vi "PDash Validate Module.vi"(8 "error in":errorcluster, 10 "Current Selection":T1, 11 "Project":refnum<class "Project.lvclass">) -> (0 "error out":errorcluster, 3 "Project Out":refnum<class "Project.lvclass">)   [LabVIEW 2020, in "Panther Dashboard.lvlib"]
doc: "Panther Dashboard DQMH UI Template"
uses:
  Panther Dashboard.lvlib
  Class/Project/Project.lvclass
  C:/GitClones/PantherDashboard/src/LabVIEW/Panther Dashboard/Class/LabVIEWItem/LabVIEWItem.lvclass
  Class/Library/Library.lvclass
  Class/VI/VI.lvclass
  Class/Library/Library.lvclass/Library.ctl
  Class/LabVIEWItem/LabVIEWItem.lvclass/LabVIEWItem.ctl
  Class/Project/Project.lvclass/Project.ctl
  Class/Library/Read Library Ref.vi
  Class/LabVIEWItem/Read Item Name.vi
  Class/Project/Read Main App Inst Ref.vi
  Class/LabVIEWItem/Read Item Path.vi
  Class/Project/Read Target Ref.vi
  Class/Project/Read Project Ref.vi
  Class/LabVIEWItem/Write Item Description.vi
  Class/Project/Write Project Ref.vi
  Class/LabVIEWItem/Write Item Name.vi
  Class/Project/Write Target Name.vi
  Class/Project/Write Target Ref.vi
  Class/Project/Write Target App Ins Ref.vi
  Class/Project/Write Main App Inst Ref.vi
  Class/LabVIEWItem/Write Item Path.vi
  Class/LabVIEWItem/Write Item Type.vi
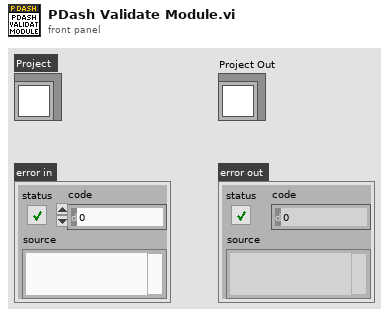
[diagram p1: front panel]
types:
  T1 = cluster{"Library":refnum<class "Library.lvclass">, "VI":refnum<class "VI.lvclass">}
  T2 = typedef "DQMH Validate Module.lvlib/Validation Result.ctl" = cluster{"Test Result":T3, "Issue Text":string, "Category Text":string, "Details Message":string, "Fixer VI":path, "Error":errorcluster, "Data for Fixer":variant, "Library":refnum<vi>, "Double Click VI":path, "Data for Double Click":variant}
  T3 = typedef "DQMH Validate Module.lvlib/Test Result.ctl" = enum16{"Pass", "Fail", "Error"}
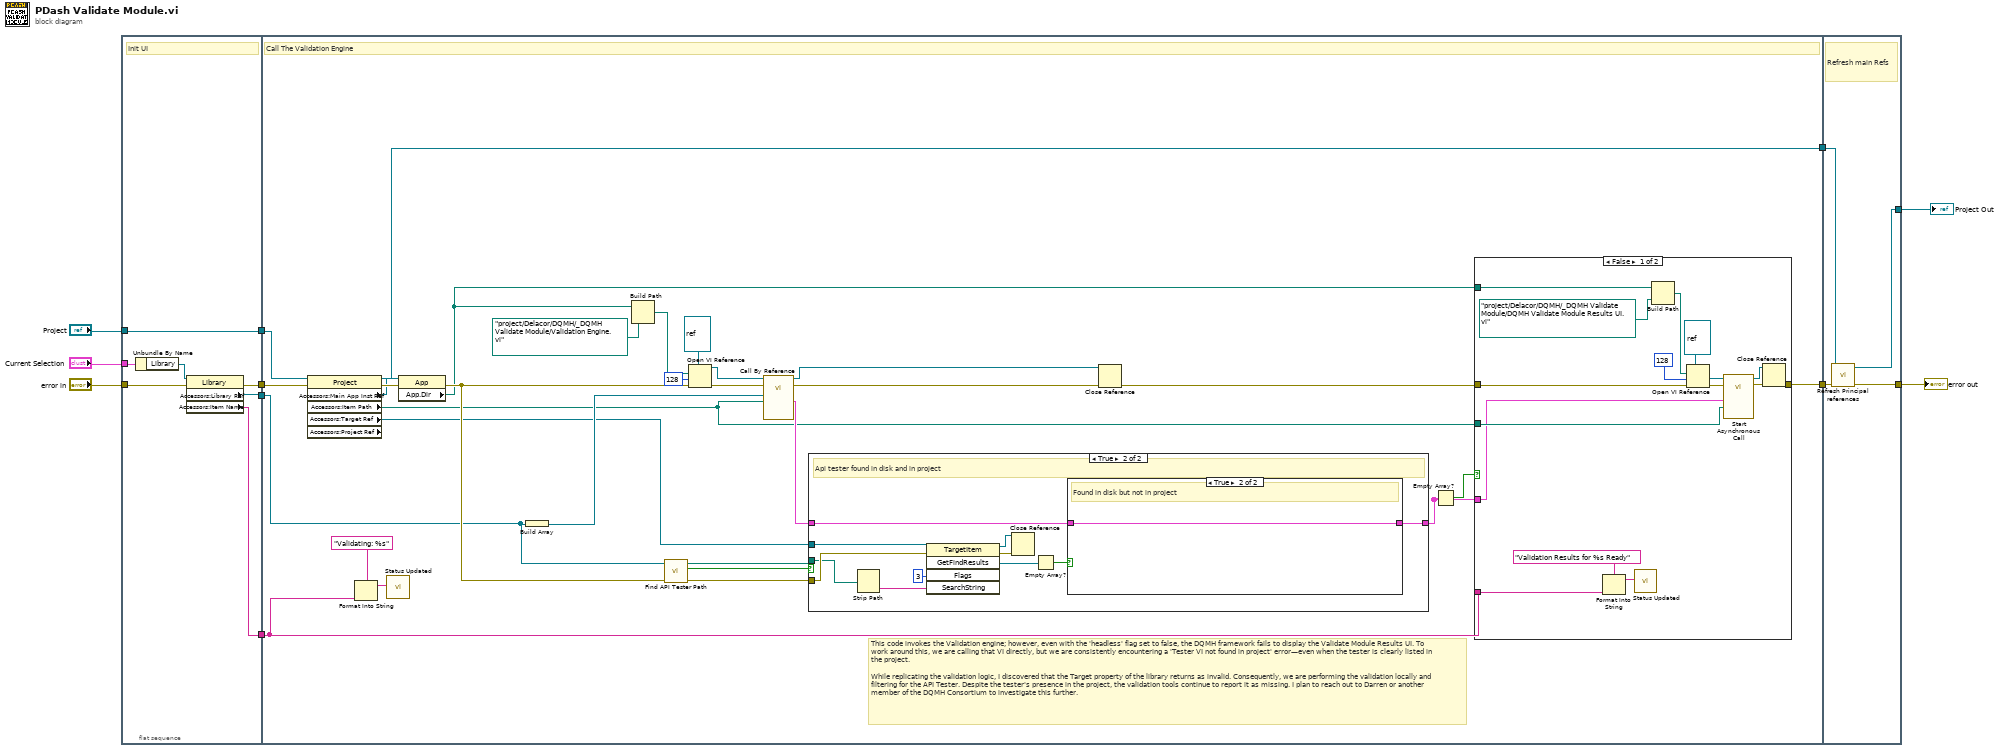
[diagram p0: block diagram]
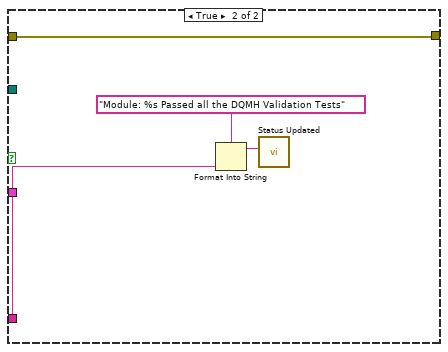
[diagram p2: hidden frame]
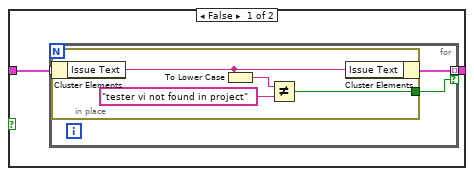
[diagram p4: hidden frame]
diagram:
  n1 = flat-sequence {
    tunnel: "Project" -> [w16]
    tunnel: [w16] -> w6
    tunnel: "error in" -> [w18]
    tunnel: [w17] -> w8
    tunnel: "Current Selection" -> [w15]
    tunnel: [w13] -> w4
    tunnel: [w12] -> w3
    tunnel: [w44] -> w11
    tunnel: w6 -> [w40]
    tunnel: w8 -> [w48]
    tunnel: w4 -> [w28]
    tunnel: w3 -> [w23]
    tunnel: [w19] -> w2
    tunnel: [w93] -> w10
    tunnel: w11 -> [w94]
    tunnel: w2 -> [w92]
    tunnel: [w91] -> w1
    frame #0 {
      # "Init UI"
      n2 = Unbundle By Name(w15) -> ("Library"=w14:refnum<class "Library.lvclass">)
      n3 = property class="Library"(reference=w14, error in=w18) -> (error out=w17:errorcluster, "Accessors:Library Ref"=w13:refnum<vi>, "Accessors:Item Name"=w12:string)  [unwired: 1 out]
    }
    frame #1 {
      # "This code invokes the Validation engine; however, even with the 'headless' flag set to false, the DQMH framework fails to display the Validate Module Results UI. To work around this, we are calling that VI directly, but we are consistently encountering a 'Tester VI not found in project' error—even when the tester is clearly listed in the project.\n\nWhile replicating the validation logic, I discovered that the Target property of the library returns as invalid. Consequently, we are performing the validation locally and filtering for the API Tester. Despite the tester's presence in the project, the validation tools continue to report it as missing. I plan to reach out to Darren or another member of the DQMH Consortium to investigate this further."
      # "Call The Validation Engine"
      n4 = property class="Project" props=["Accessors:Main App Inst Ref", "Accessors:Item Path", "Accessors:Target Ref", "Accessors:Project Ref"](reference=w40, error in=w48) -> (reference out=w19:refnum<class "Project.lvclass">, error out=w47:errorcluster, "Accessors:Main App Inst Ref"=w39:refnum<vi>, "Accessors:Item Path"=w26:path, "Accessors:Target Ref"=w20:refnum<vi>)  [unwired: 1 out]
      n5 = Format Into String(format string="Validating: %s" ("Status"), w23) -> (resulting string=w34:string)  [unwired: 2 in, 1 out]
      n6 = call "Status Updated.vi"("Status"=w34) -> ()  [unwired: 10 in, 1 out]
      n7 = property class="App"(reference=w39, error in=w47) -> (error out=w42:errorcluster, "App.Dir"=w31:path)  [unwired: 1 out]
      n8 = Build Array(w28) -> (w35:refnum<vi>[])
      n9 = Build Path(base path=w31, name or relative path=path "project/Delacor/DQMH/_DQMH Validate Module/Validation Engine.vi") -> (appended path=w38:path)
      n10 = call "Find API Tester Path.vi"("error in"=w42, "DQMH Library Ref"=w28) -> ("error out"=w41:errorcluster, "Api tester found?"=w22:bool, "API Tester Path"=w21:path)  [unwired: 7 in]
      n11 = Open VI Reference(type specifier VI Refnum (for type only)=refnum<vi> refnum, vi path=w38, options=128, error in (no error)=w42) -> (vi reference=w32:refnum<vi>, error out=w43:errorcluster)  [unwired: 2 in]
      n12 = call-by-ref "?"(reference=w32, error in=w43, "Project Path"=w26, "Libraries in"=w35) -> (reference out=w30:refnum<vi>, error out=w46:errorcluster, "Validation Results"=w27:T2[])  [unwired: 6 in, 3 out]
      n13 = case shown="True" w22 {
        tunnel: w27 -> [w69 w78]
        tunnel: [w69 w77] -> w25
        tunnel: w41 -> [_ w79]
        tunnel: w21 -> [_ w73]
        tunnel: w20 -> [_ w72]
        frame False {
          # "Api Tester Not found in project"
        }
        frame True {
          # "Api tester found in disk and in project"
          n14 = Strip Path(path=w73) -> (name=w75:string)  [unwired: 1 out]
          n15 = invoke class="TargetItem" method="GetFindResults"(reference=w72, error in=w79, "Flags"=3, "SearchString"=w75) -> (reference out=w70:refnum<vi>, error out=w80:errorcluster, "GetFindResults"=w74:refnum<vi>[])  [unwired: 1 in, 2 out]
          n16 = Close Reference(reference=w70, error in (no error)=w80) -> ()  [unwired: 1 out]
          n17 = Empty Array?(array=w74) -> (empty?=w71:bool)
          n18 = case shown="True" w71 {
            tunnel: w78 -> [w82 w90]
            tunnel: [w81 w90] -> w77
            frame False {
              n19 = for {
                tunnel: w82 -> [w85] mode=indexing
                tunnel: [w84] -> w81 mode=indexing if=w83
                n20 = in-place {
                  in-place-border: [w87] -> w83
                  n21 = in-place-cluster #1(w85) -> ("Issue Text"=w88:string)
                  n22 = To Lower Case(string=w88) -> (all lower case string=w86:string)
                  n23 = Not Equal?(x=w86, y="tester vi not found in project") -> (x != y?=w87:bool)
                  n24 = in-place-cluster #1("Issue Text"=w88) -> (w84:T2)
                }
              }
            }
            frame True {
              # "Found in disk but not in project"
            }
          }
        }
      }
      n25 = Close Reference(reference=w30, error in (no error)=w46) -> (error out=w45:errorcluster)
      n26 = Empty Array?(array=w25) -> (empty?=w24:bool)
      n27 = case shown="False" w24 {
        tunnel: w45 -> [w62 w68]
        tunnel: [w61 w68] -> w44
        tunnel: w31 -> [w59 _]
        tunnel: w26 -> [w53 _]
        tunnel: w25 -> [w52 _]
        tunnel: w23 -> [w49 w65]
        frame False {
          n28 = Format Into String(format string="Validation Results for %s Ready" ("Status"), w49) -> (resulting string=w50:string)  [unwired: 2 in, 1 out]
          n29 = call "Status Updated.vi"("Status"=w50) -> ()  [unwired: 10 in, 1 out]
          n30 = Build Path(base path=w59, name or relative path=path "project/Delacor/DQMH/_DQMH Validate Module/DQMH Validate Module Results UI.vi") -> (appended path=w55:path)
          n31 = Open VI Reference(type specifier VI Refnum (for type only)=refnum<vi> refnum, vi path=w55, options=128, error in (no error)=w62) -> (vi reference=w57:refnum<vi>, error out=w63:errorcluster)  [unwired: 2 in]
          n32 = call-by-ref "Start Asynchronous Call"(reference=w57, error in=w63, "Project Path"=w53, "Validation Results"=w52) -> (reference out=w58:refnum<vi>, error out=w64:errorcluster)  [unwired: 9 in, 1 out]
          n33 = Close Reference(reference=w58, error in (no error)=w64) -> (error out=w61:errorcluster)
        }
        frame True {
          n34 = Format Into String(format string="Module: %s Passed all the DQMH Validation Tests" ("Status"), w65) -> (resulting string=w67:string)  [unwired: 2 in, 1 out]
          n35 = call "Status Updated.vi"("Status"=w67) -> ()  [unwired: 10 in, 1 out]
        }
      }
    }
    frame #2 {
      # "Refresh main Refs"
      n36 = call "Refresh Principal references.vi"("error in"=w94, "Project in"=w92) -> ("error out"=w93:errorcluster, "Project out"=w91:refnum<class "Project.lvclass">)  [unwired: 8 in]
    }
  }
  "error out" <- w10
  "Project Out" <- w1
